vi "RedistributeArmPathPointsVariable.vi"(1 "DesiredPointSpacing":dbl[](array[numeric]), 2 "ArmPathIn":T1[](array[typedef]), 3 "IndexedPathLength":dbl[](array[numeric])) -> (0 "ArmPathOut":T1[](array[typedef]))   [LabVIEW 2018]
uses:
  TypeDefs/ArmCoordinate.ctl
  ArgosLib/ArgosLib.lvlib
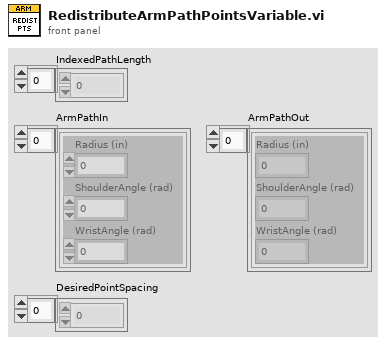
[diagram p1: front panel]
types:
  T1 = typedef "ArmCoordinate.ctl" = cluster{"Radius (in)":dbl, "ShoulderAngle (rad)":dbl, "WristAngle (rad)":dbl}
  T2 = typedef "ArgosLib.lvlib/Point2D.ctl" = cluster{"X (in)":dbl, "Y (in)":dbl, "Wrist Angle (rad)":dbl}
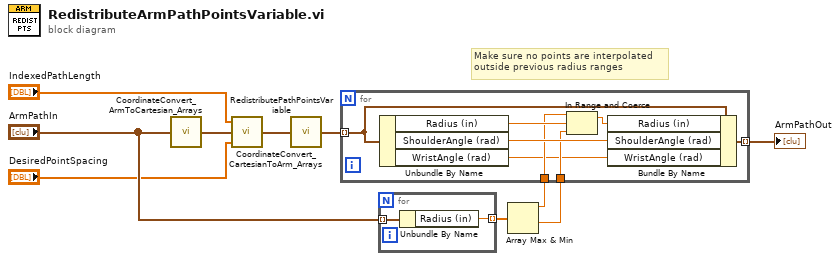
[diagram p0: block diagram]
diagram:
  # "Make sure no points are interpolated\noutside previous radius ranges"
  n1 = call "CoordinateConvert_ArmToCartesian_Arrays.vi"("ArmCoordinates"="ArmPathIn") -> ("XYPoints"=w3:T2[])
  n2 = call "RedistributePathPointsVariable.vi"("DesiredPointSpacing"="DesiredPointSpacing", "PathIn"=w3, "IndexedPathLength"="IndexedPathLength") -> ("PathOut"=w4:T2[])
  n3 = call "CoordinateConvert_CartesianToArm_Arrays.vi"("XYPoints"=w4) -> ("ArmCoordinates"=w8:T1[])
  n4 = for {
    tunnel: "ArmPathIn" -> [w12] mode=indexing
    tunnel: [w11] -> w10 mode=indexing
    n5 = Unbundle By Name(w12) -> ("Radius (in)"=w11:dbl)
  }
  n6 = Array Max & Min(array=w10) -> (max value=w6:dbl, min value=w5:dbl)  [unwired: 2 out]
  n7 = for {
    tunnel: w8 -> [w19] mode=indexing
    tunnel: [w20] -> w7 mode=indexing
    tunnel: w6 -> [w15]
    tunnel: w5 -> [w14]
    n8 = Unbundle By Name(w19) -> ("Radius (in)"=w16:dbl, "ShoulderAngle (rad)"=w18:dbl, "WristAngle (rad)"=w13:dbl)
    n9 = In Range and Coerce(upper limit=w15, x=w16, lower limit=w14) -> (coerced(x)=w17:dbl)  [unwired: 1 out]
    n10 = Bundle By Name(cluster=w19, "Radius (in)"=w17, "ShoulderAngle (rad)"=w18, "WristAngle (rad)"=w13) -> (w20:T1)
  }
  "ArmPathOut" <- w7
